vi "NI-DP_GetDeviceInfo.vi"(5 "RX Port No.":u16, 6 "timeout [ms]":u32, 7 "IP to write to":string, 8 "error in (no error)":errorcluster, 9 "Device Mac Address (hex)":string="\u0000\u0000\u0000\u0000\u0000\u0000", 11 "UDP Network Connection in":refnum<k16>) -> (0 "error out":errorcluster, 3 "UDP Network Connection out":refnum<k16>, 4 "RxData":T1 {"Command" items=["0x01: Get Type & Hostname"=1, "0x03: Set IP 1"=3, "0x04: Set IP 2"=4, "0x08: Acknowledge"=8, "0x0A: Reboot"=10, "0x20: ???"=32, "0x21: ???"=33, "0xF2: System State"=242, "0xF4: System Details"=244]})   [LabVIEW 2014, in "hse-network.lvlib"]
doc: "____\nHAMPEL SOFTWARE ENGINEERING v0.7.0 (2018-07-16 18:12)"
uses:
  hse-network.lvlib
  NI-DP__MessageStructure.ctl
  NI-DP__Commands.ctl
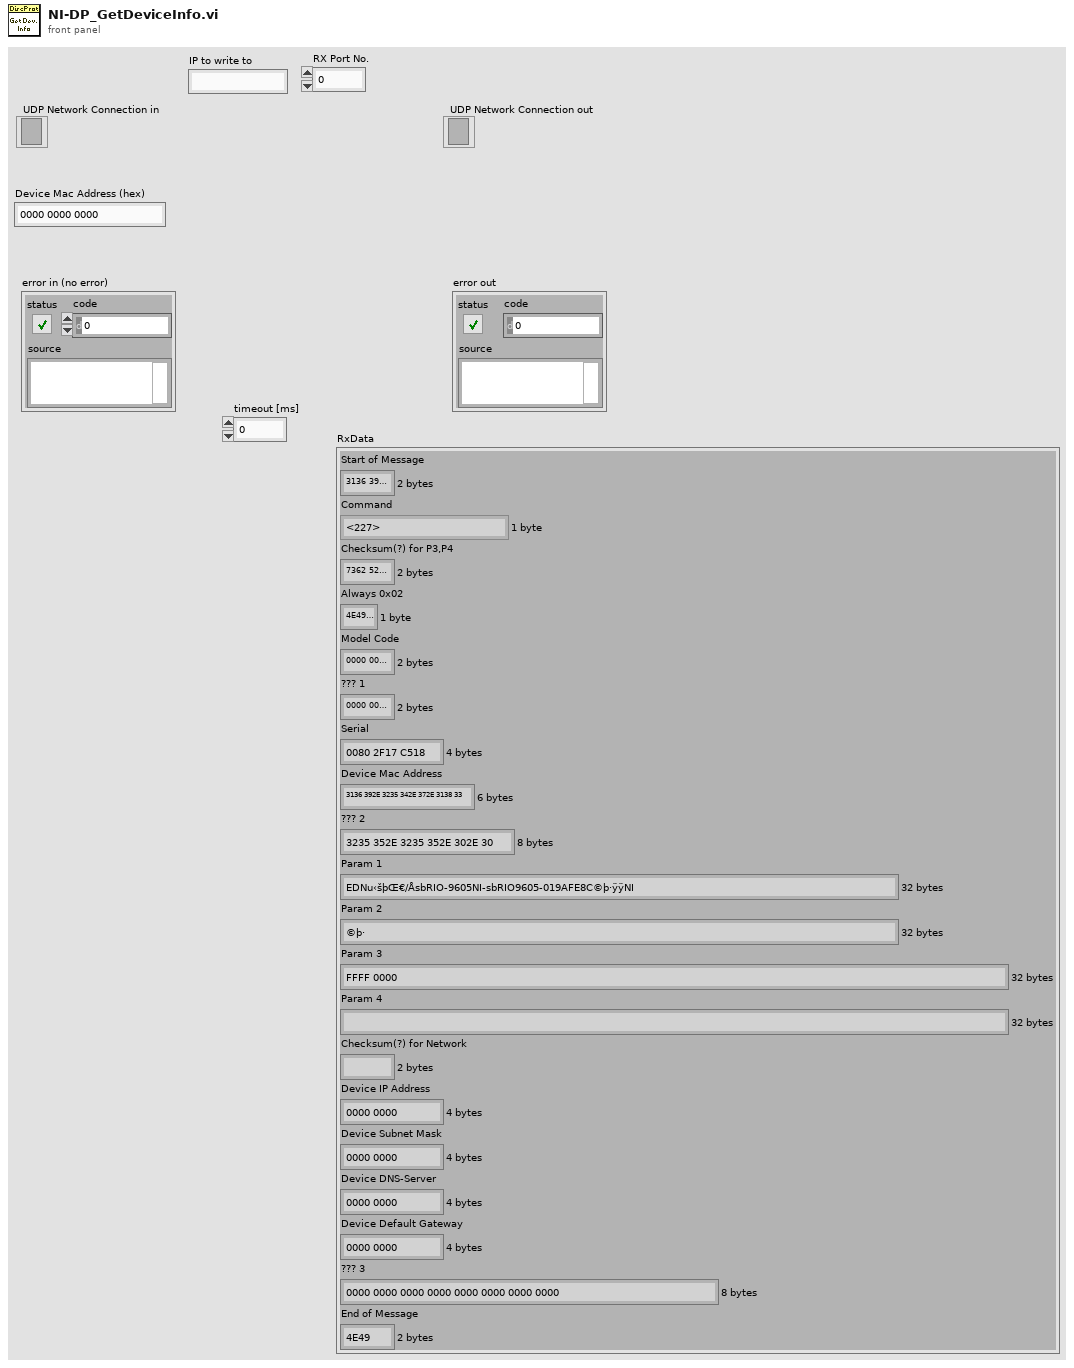
[diagram p1: front panel]
types:
  T1 = typedef "hse-network.lvlib/NI-DP__MessageStructure.ctl" = cluster{"Start of Message":string, "Command":T2, "Checksum(?) for P3,P4":string, "Always 0x02":string, "Model Code":string, "??? 1":string, "Serial":string, "Device Mac Address":string, "??? 2":string, "Param 1":string, "Param 2":string, "Param 3":string, "Param 4":string, "Checksum(?) for Network":string, "Device IP Address":string, "Device Subnet Mask":string, "Device DNS-Server":string, "Device Default Gateway":string, "??? 3":string, "End of Message":string}
  T2 = typedef "hse-network.lvlib/NI-DP__Commands.ctl" = u8
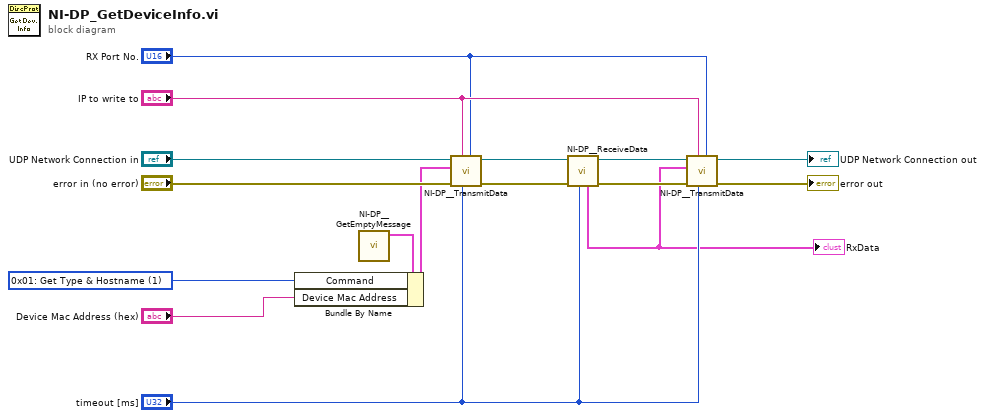
[diagram p0: block diagram]
diagram:
  w13 = T2 1 items=["0x01: Get Type & Hostname"=1, "0x03: Set IP 1"=3, "0x04: Set IP 2"=4, "0x08: Acknowledge"=8, "0x0A: Reboot"=10, "0x20: ???"=32, "0x21: ???"=33, "0xF2: System State"=242, "0xF4: System Details"=244] ("Command")
  n1 = call "NI-DP__GetEmptyMessage.vi"() -> ("NI-DP__EmptyMessage"=w9:T1)  [unwired: 11 in]
  n2 = Bundle By Name(cluster=w9, "Command"=w13, "Device Mac Address"="Device Mac Address (hex)") -> (w14:T1)
  n3 = call "NI-DP__TransmitData.vi"("Port to write to"="RX Port No.", "timeout ms"="timeout [ms]", "IP to write to"="IP to write to", "error in"="error in (no error)", "UDP-NI__Message"=w14, "UDP Network Connection in"="UDP Network Connection in") -> ("error out"=w12:errorcluster, "UDP Network Connection out"=w11:refnum<k16>)  [unwired: 4 in]
  n4 = call "NI-DP__ReceiveData.vi"("timeout [ms]"="timeout [ms]", "error in"=w12, "UDP Network Connection in"=w11) -> ("error out"=w5:errorcluster, "UDP Network Connection out"=w4:refnum<k16>, "UDP-NI Message"=w1:T1)  [unwired: 3 in, 3 out]
  "RxData" <- w1
  n5 = call "NI-DP__TransmitData.vi"("Port to write to"="RX Port No.", "timeout ms"="timeout [ms]", "IP to write to"="IP to write to", "error in"=w5, "UDP-NI__Message"=w1, "UDP Network Connection in"=w4) -> ("error out"=→"error out":errorcluster, "UDP Network Connection out"=→"UDP Network Connection out":refnum<k16>)  [unwired: 4 in]
